vi "加速度_波形指标.vi"(10 "均方根值":dbl, 11 "信号X":dbl[](array[numeric])) -> (3 "波形指标":dbl)   [LabVIEW 2014]
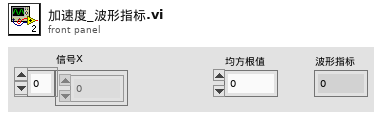
[diagram p1: front panel]
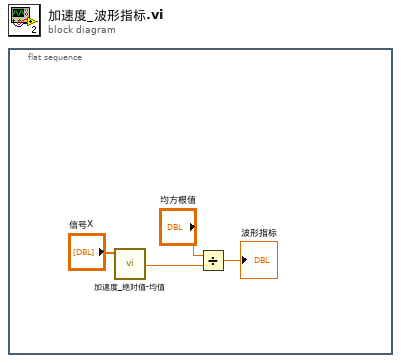
[diagram p0: block diagram]
diagram:
  n1 = flat-sequence {
    frame #0 {
      n2 = call "加速度_绝对值-均值.vi"("信号X"="信号X") -> ("均值"=w2:dbl)  [unwired: 10 in]
      n3 = Divide(x="均方根值", y=w2) -> (x/y=→"波形指标":dbl)
    }
  }
